vi "Show Dendrites.vi"(8 "error in (no error)":errorcluster, 10 "LUT1":cluster{u16, u16}(slide)={0, 4095} caption="Slide" scale=0.0..4095.0, 11 "Input Image":T1(plugin-control)) -> (0 "error out":errorcluster, 1 "most Verital":T2, 2 "most horizontal":T2, 3 "Reference Screen":T1(plugin-control), 4 "height":dbl, 5 "width":dbl)   [LabVIEW 2020]
uses:
  <vilib>/vision/NI_Vision_Development_Module.lvlib
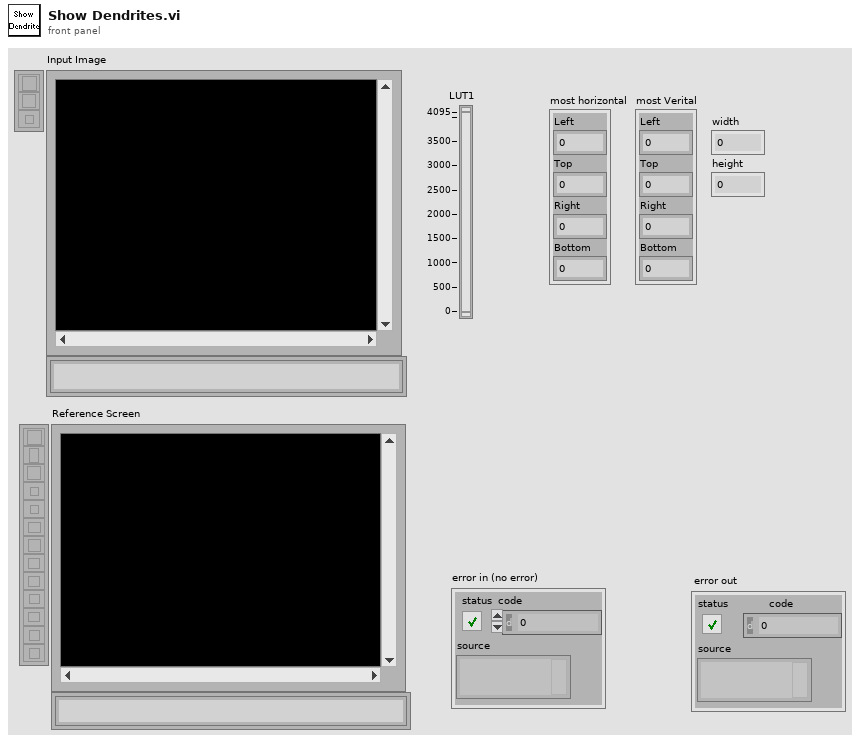
[diagram p1: front panel]
types:
  T1 = typedef "IMAQ Image.ctl" = refnum<image>
  T2 = cluster{"Left":i32, "Top":i32, "Right":i32, "Bottom":i32}
  T3 = typedef "Image Type" = u32
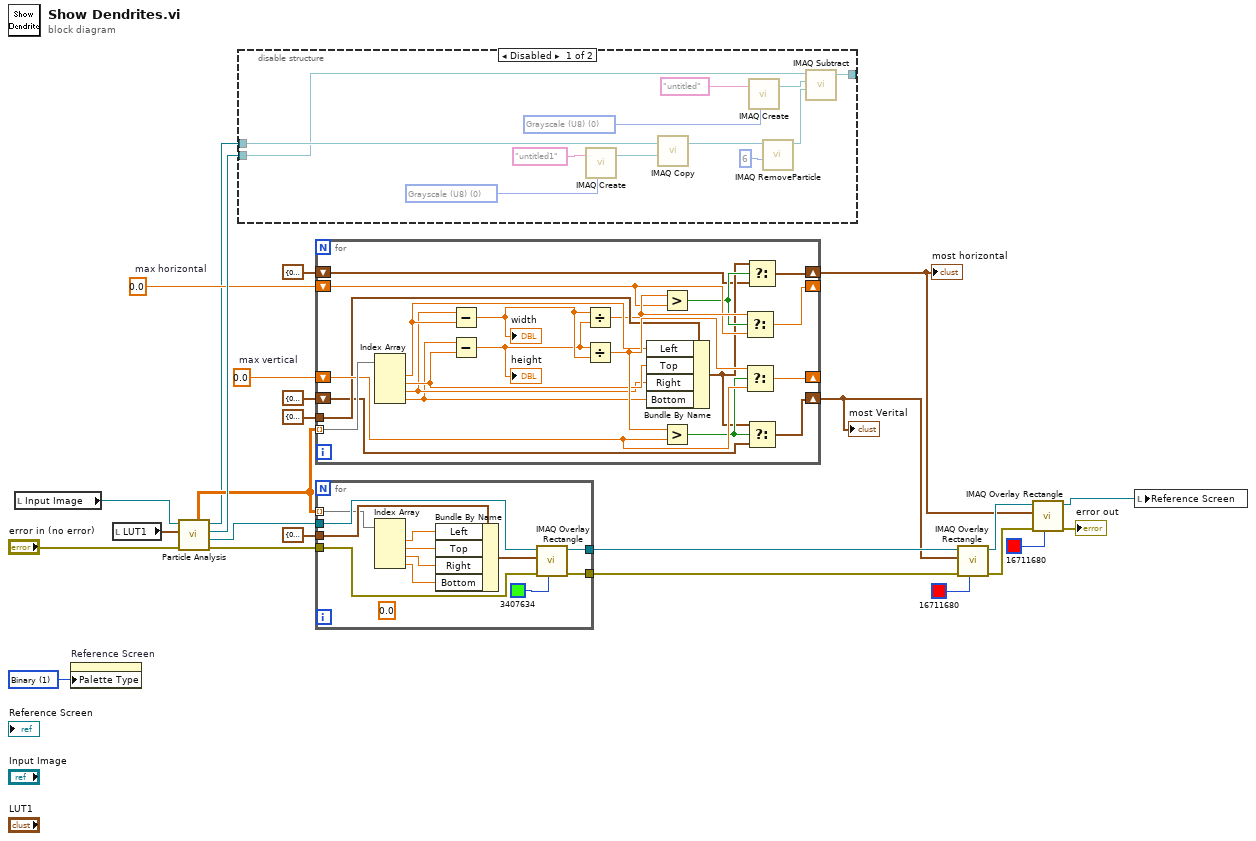
[diagram p0: block diagram]
diagram:
  w17 = 0.0  # max horizontal
  w18 = 0.0  # max vertical
  w23 = u32 1 items=["Grayscale", "Binary", "Gradient", "Rainbow", "Temperature", "User Defined"] ("Palette:Palette Type")
  n1 = local read "Input Image"() -> (w25:T1)
  n2 = property on="Reference Screen" class="ImageControl"("Palette Type"=w23) -> ()  [unwired: 2 in, 2 out]
  n3 = local read "LUT1"() -> (w24:cluster{u16, u16})
  n4 = call "Particle Analysis.vi"("error in (no error)"="error in (no error)", "LUT1"=w24, "Image in"=w25) -> ("error out"=w2:errorcluster, "Image Out"=w22:T1, "Image Dst Out 2"=w20:T1, "Image Dst Out 1"=w4:T1, "Particle Measurements (Pixels)"=w19:dbl[][])  [unwired: 4 in]
  n5 = disable-structure shown="Disabled" {
    disable-tunnel: w4 -> [w37 _]
    disable-tunnel: w20 -> [w36 _]
    disable-tunnel: [w35 _] -> _
    frame Disabled {
      w28 = T3 0 items=["Grayscale (U8)", "Grayscale (I16)", "Grayscale (SGL)", "Complex (CSG)", "RGB (U32)", "HSL (U32)", "RGB (U64)", "Grayscale (U16)"] ("Image Type")
      w33 = T3 0 items=["Grayscale (U8)", "Grayscale (I16)", "Grayscale (SGL)", "Complex (CSG)", "RGB (U32)", "HSL (U32)", "RGB (U64)", "Grayscale (U16)"] ("Image Type")
      n6 = call "IMAQ Create"("Image Name"="untitled1", "Image Type"=w28) -> ("New Image"=w27:T1)  [unwired: 3 in, 1 out]
      n7 = call "IMAQ Copy"("Image Dst"=w27, "Image Src"=w37) -> ("Image Dst Out"=w26:T1)  [unwired: 4 in, 1 out]
      n8 = call "IMAQ Create"("Image Name"="untitled", "Image Type"=w33) -> ("New Image"=w31:T1)  [unwired: 3 in, 1 out]
      n9 = call "IMAQ RemoveParticle"("Number of Erosion"=6, "Image Src"=w26) -> ("Image Dst Out"=w30:T1)  [unwired: 5 in, 4 out]
      n10 = call "IMAQ Subtract"("Image Src A"=w36, "Image Dst"=w31, "Image Src B"=w30) -> ("Image Dst Out"=w35:T1)  [unwired: 4 in, 1 out]
    }
    frame Enabled {
    }
  }
  n11 = for {
    tunnel: w19 -> [w58] mode=indexing
    shift-right: [w53] -> _
    shift-left: w18 -> [w54]
    shift-right: [w42] -> _
    shift-left: w17 -> [w43]
    tunnel: T2 {"Left"=0, "Top"=0, "Right"=0, "Bottom"=0} ("Rectangle") -> [w48]
    shift-right: [w46] -> w12
    shift-left: T2 {"Left"=0, "Top"=0, "Right"=0, "Bottom"=0} ("Rectangle") -> [w45]
    shift-right: [w39] -> w9
    shift-left: T2 {"Left"=0, "Top"=0, "Right"=0, "Bottom"=0} ("Rectangle") -> [w38]
    n12 = Index Array(array=w58) -> (element #1=w52:dbl, element #2=w51:dbl, element #3=w50:dbl, element #4=w49:dbl)  [unwired: 4 in]
    n13 = Subtract(x=w50, y=w52) -> (x-y=w57:dbl)
    "width" <- w57
    n14 = Subtract(x=w49, y=w51) -> (x-y=w56:dbl)
    "height" <- w56
    n15 = Divide(x=w57, y=w56) -> (x/y=w44:dbl)
    n16 = Divide(x=w56, y=w57) -> (x/y=w55:dbl)
    n17 = Bundle By Name(cluster=w48, "Left"=w52, "Top"=w51, "Right"=w50, "Bottom"=w49) -> (w40:T2)
    n18 = Greater?(x=w44, y=w43) -> (0:w41:bool)
    n19 = Greater?(x=w55, y=w54) -> (0:w47:bool)
    n20 = Select(t=w44, s=w41, f=w43) -> (s? t:f=w42:dbl)
    n21 = Select(t=w55, s=w47, f=w54) -> (s? t:f=w53:dbl)
    n22 = Select(t=w40, s=w41, f=w38) -> (s? t:f=w39:T2)
    n23 = Select(t=w40, s=w47, f=w45) -> (s? t:f=w46:T2)
  }
  "most Verital" <- w12
  "most horizontal" <- w9
  n24 = for {
    tunnel: [w61] -> w13
    tunnel: w22 -> [w69]
    tunnel: w19 -> [w67] mode=indexing
    tunnel: T2 {"Left"=0, "Top"=0, "Right"=0, "Bottom"=0} ("Rectangle") -> [w68]
    tunnel: [w60] -> w6
    tunnel: w2 -> [w59]
    (unwired) 0.0 ("Rotation")
    n25 = Index Array(array=w67) -> (element #1=w65:dbl, element #2=w64:dbl, element #3=w63:dbl, element #4=w62:dbl)  [unwired: 4 in]
    n26 = Bundle By Name(cluster=w68, "Left"=w65, "Top"=w64, "Right"=w63, "Bottom"=w62) -> (w66:T2)
    n27 = call "IMAQ Overlay Rectangle"("Color"=u32 3407634 ("Text Color (black)"), "error in (no error)"=w59, "Rectangle"=w66, "Image"=w69) -> ("error out"=w60:errorcluster, "Image Out"=w61:T1)  [unwired: 6 in]
  }
  n28 = call "IMAQ Overlay Rectangle"("Color"=u32 16711680, "error in (no error)"=w6, "Rectangle"=w12, "Image"=w13) -> ("error out"=w5:errorcluster, "Image Out"=w10:T1)  [unwired: 6 in]
  n29 = call "IMAQ Overlay Rectangle"("Color"=u32 16711680, "error in (no error)"=w5, "Rectangle"=w9, "Image"=w10) -> ("error out"=→"error out":errorcluster, "Image Out"=w7:T1)  [unwired: 6 in]
  n30 = local write "Reference Screen"(w7) -> ()
